vi "BCU诊断标定.vi"(8 "CAN端口":u16(ring), 9 "设备索引号":u16(ring), 10 "CAN卡类型":u32(ring)=21, 11 "Myindex":dbl=1.0) -> (3 "成功":bool)   [LabVIEW 2013] (continued)
                n1426 = global read "功能码全局.vi" "24"() -> (w1888:bool[])
                n1427 = global read "功能码全局.vi" "23"() -> (w1889:bool[])
                n1428 = Index Array(array=w1888) -> (element #3=w1878:bool, element #4=w1877:bool, element #5=w1876:bool, element #6=w1875:bool, element #7=w1874:bool, element #8=w1873:bool)  [unwired: 8 in, 2 out]
                n1429 = Index Array(array=w1889) -> (element #3=w1887:bool, element #4=w1886:bool, element #5=w1885:bool, element #6=w1884:bool, element #7=w1883:bool, element #8=w1882:bool)  [unwired: 8 in, 2 out]
                n1430 = Build Array(w1878, w1877, w1876, w1875, w1874, w1873) -> (w1879:bool[])
                n1431 = Build Array(w1887, w1886, w1885, w1884, w1883, w1882) -> (w1881:bool[])
                n1432 = And Array Elements(Boolean array=w1879) -> (logical AND=w1872:bool)
                n1433 = And Array Elements(Boolean array=w1881) -> (logical AND=w1880:bool)
                n1434 = Not(x=w1871) -> (.not. x?=w1895:bool)
              }
              frame "电池包信息1" {
                w1900 = 2
                w1908 = 2
                w1899 = 2
                w1897 = FALSE ("1 6")
                n1435 = Select(t=0, s=w1905, f=1) -> (s? t:f=w1898:i32)
                n1436 = property on="串联数" class="DigNum (严格)"("Disabled"=w1898) -> ()  [unwired: 2 in, 2 out]
                n1437 = property on="并联数" class="DigNum (严格)"("Disabled"=w1898) -> ()  [unwired: 2 in, 2 out]
                n1438 = property on="电池厂家" class="DigNum (严格)"("Disabled"=w1898) -> ()  [unwired: 2 in, 2 out]
                n1439 = property on="电池类型" class="DigNum (严格)"("Disabled"=w1898) -> ()  [unwired: 2 in, 2 out]
                n1440 = property on="额定能量" class="DigNum (严格)"("Disabled"=w1898) -> ()  [unwired: 2 in, 2 out]
                n1441 = property on="额定容量" class="DigNum (严格)"("Disabled"=w1898) -> ()  [unwired: 2 in, 2 out]
                n1442 = property on="实际容量" class="DigNum (严格)"("Disabled"=w1898) -> ()  [unwired: 2 in, 2 out]
                n1443 = property on="电池组信息" class="Clust (严格)"("Disabled"=w1898) -> ()  [unwired: 2 in, 2 out]
                n1444 = property on="生产日期" class="Str"("DisabledEnum"=w1898) -> ()  [unwired: 2 in, 2 out]
                n1445 = property on="车牌号" class="Str"("DisabledEnum"=w1899) -> ()  [unwired: 2 in, 2 out]
                n1446 = property on="产权标识" class="DigNum (严格)"("Disabled"=w1898) -> ()  [unwired: 2 in, 2 out]
                n1447 = property on="应用车型" class="DigNum (严格)"("Disabled"=w1898) -> ()  [unwired: 2 in, 2 out]
                n1448 = property on="额定总压" class="DigNum (严格)"("Disabled"=w1898) -> ()  [unwired: 2 in, 2 out]
                n1449 = property on="电池包序号" class="DigNum (严格)"("DisabledEnum"=w1898) -> ()  [unwired: 2 in, 2 out]
                n1450 = property on="电池包组号" class="DigNum (严格)"("DisabledEnum"=w1899) -> ()  [unwired: 2 in, 2 out]
                n1451 = property on="最大允许单体电压" class="DigNum (严格)"("Disabled"=w1908) -> ()  [unwired: 2 in, 2 out]
                n1452 = property on="最大允许总电压" class="DigNum (严格)"("Disabled"=w1908) -> ()  [unwired: 2 in, 2 out]
                n1453 = property on="最大允许温度" class="DigNum (严格)"("Disabled"=w1908) -> ()  [unwired: 2 in, 2 out]
                n1454 = property on="最小允许温度" class="DigNum (严格)"("Disabled"=w1908) -> ()  [unwired: 2 in, 2 out]
                n1455 = property on="最大允许充电电流" class="DigNum (严格)"("Disabled"=w1908) -> ()  [unwired: 2 in, 2 out]
                n1456 = property on="最小允许充电电流" class="DigNum (严格)"("Disabled"=w1908) -> ()  [unwired: 2 in, 2 out]
                n1457 = property on="最小允许单体电压" class="DigNum (严格)"("Disabled"=w1908) -> ()  [unwired: 2 in, 2 out]
                n1458 = property on="电流步长" class="DigNum (严格)"("Disabled"=w1908) -> ()  [unwired: 2 in, 2 out]
                n1459 = property on="SOC" class="DigNum (严格)"("Disabled"=w1908) -> ()  [unwired: 2 in, 2 out]
                n1460 = property on="充电总安时" class="DigNum (严格)"("Disabled"=w1908) -> ()  [unwired: 2 in, 2 out]
                n1461 = property on="放电总安时" class="DigNum (严格)"("Disabled"=w1908) -> ()  [unwired: 2 in, 2 out]
                n1462 = property on="放空次数" class="DigNum (严格)"("DisabledEnum"=w1900) -> ()  [unwired: 2 in, 2 out]
                n1463 = property on="充满次数" class="DigNum (严格)"("DisabledEnum"=w1900) -> ()  [unwired: 2 in, 2 out]
                n1464 = property on="充电次数" class="DigNum (严格)"("DisabledEnum"=w1900) -> ()  [unwired: 2 in, 2 out]
                n1465 = global read "功能码全局.vi" "24"() -> (w1903:bool[])
                n1466 = global read "功能码全局.vi" "23"() -> (w1904:bool[])
                n1467 = Index Array(array=w1903) -> (element #3=w1901:bool)  [unwired: 8 in, 7 out]
                n1468 = Index Array(array=w1904) -> (element #3=w1902:bool)  [unwired: 8 in, 7 out]
                n1469 = Not(x=w1897) -> (.not. x?=w1909:bool)
              }
              frame "电池包组号" {
                w1914 = 2
                w1913 = 2
                w1923 = 2
                w1915 = 2
                w1924 = 2
                w1911 = FALSE ("1 6")
                n1470 = property on="串联数" class="DigNum (严格)"("Disabled"=w1924) -> ()  [unwired: 2 in, 2 out]
                n1471 = property on="并联数" class="DigNum (严格)"("Disabled"=w1924) -> ()  [unwired: 2 in, 2 out]
                n1472 = property on="电池厂家" class="DigNum (严格)"("Disabled"=w1924) -> ()  [unwired: 2 in, 2 out]
                n1473 = property on="电池类型" class="DigNum (严格)"("Disabled"=w1924) -> ()  [unwired: 2 in, 2 out]
                n1474 = property on="额定能量" class="DigNum (严格)"("Disabled"=w1924) -> ()  [unwired: 2 in, 2 out]
                n1475 = property on="额定容量" class="DigNum (严格)"("Disabled"=w1924) -> ()  [unwired: 2 in, 2 out]
                n1476 = property on="实际容量" class="DigNum (严格)"("Disabled"=w1924) -> ()  [unwired: 2 in, 2 out]
                n1477 = Select(t=0, s=w1920, f=1) -> (s? t:f=w1912:i32)
                n1478 = property on="生产日期" class="Str"("DisabledEnum"=w1914) -> ()  [unwired: 2 in, 2 out]
                n1479 = property on="电池包序号" class="DigNum (严格)"("DisabledEnum"=w1914) -> ()  [unwired: 2 in, 2 out]
                n1480 = property on="车牌号" class="Str"("DisabledEnum"=w1914) -> ()  [unwired: 2 in, 2 out]
                n1481 = property on="电池包组号" class="DigNum (严格)"("DisabledEnum"=w1912) -> ()  [unwired: 2 in, 2 out]
                n1482 = property on="电池组信息" class="Clust (严格)"("Disabled"=w1912) -> ()  [unwired: 2 in, 2 out]
                n1483 = property on="产权标识" class="DigNum (严格)"("Disabled"=w1915) -> ()  [unwired: 2 in, 2 out]
                n1484 = property on="应用车型" class="DigNum (严格)"("Disabled"=w1915) -> ()  [unwired: 2 in, 2 out]
                n1485 = property on="额定总压" class="DigNum (严格)"("Disabled"=w1915) -> ()  [unwired: 2 in, 2 out]
                n1486 = property on="放空次数" class="DigNum (严格)"("DisabledEnum"=w1913) -> ()  [unwired: 2 in, 2 out]
                n1487 = property on="充满次数" class="DigNum (严格)"("DisabledEnum"=w1913) -> ()  [unwired: 2 in, 2 out]
                n1488 = property on="充电次数" class="DigNum (严格)"("DisabledEnum"=w1913) -> ()  [unwired: 2 in, 2 out]
                n1489 = property on="最大允许单体电压" class="DigNum (严格)"("Disabled"=w1923) -> ()  [unwired: 2 in, 2 out]
                n1490 = property on="最大允许总电压" class="DigNum (严格)"("Disabled"=w1923) -> ()  [unwired: 2 in, 2 out]
                n1491 = property on="最大允许温度" class="DigNum (严格)"("Disabled"=w1923) -> ()  [unwired: 2 in, 2 out]
                n1492 = property on="最小允许温度" class="DigNum (严格)"("Disabled"=w1923) -> ()  [unwired: 2 in, 2 out]
                n1493 = property on="最大允许充电电流" class="DigNum (严格)"("Disabled"=w1923) -> ()  [unwired: 2 in, 2 out]
                n1494 = property on="最小允许充电电流" class="DigNum (严格)"("Disabled"=w1923) -> ()  [unwired: 2 in, 2 out]
                n1495 = property on="最小允许单体电压" class="DigNum (严格)"("Disabled"=w1923) -> ()  [unwired: 2 in, 2 out]
                n1496 = property on="电流步长" class="DigNum (严格)"("Disabled"=w1923) -> ()  [unwired: 2 in, 2 out]
                n1497 = property on="SOC" class="DigNum (严格)"("Disabled"=w1923) -> ()  [unwired: 2 in, 2 out]
                n1498 = property on="充电总安时" class="DigNum (严格)"("Disabled"=w1923) -> ()  [unwired: 2 in, 2 out]
                n1499 = property on="放电总安时" class="DigNum (严格)"("Disabled"=w1923) -> ()  [unwired: 2 in, 2 out]
                n1500 = global read "功能码全局.vi" "24"() -> (w1918:bool[])
                n1501 = global read "功能码全局.vi" "23"() -> (w1919:bool[])
                n1502 = Index Array(array=w1918) -> (element #3=w1916:bool)  [unwired: 8 in, 7 out]
                n1503 = Index Array(array=w1919) -> (element #3=w1917:bool)  [unwired: 8 in, 7 out]
                n1504 = Not(x=w1911) -> (.not. x?=w1925:bool)
              }
              frame "充放电安时" {
                w1929 = 2
                w1928 = 2
                w1938 = 2
                w1939 = 2
                w1941 = 2
                w1927 = FALSE ("1 6")
                n1505 = property on="串联数" class="DigNum (严格)"("Disabled"=w1941) -> ()  [unwired: 2 in, 2 out]
                n1506 = property on="并联数" class="DigNum (严格)"("Disabled"=w1941) -> ()  [unwired: 2 in, 2 out]
                n1507 = property on="电池厂家" class="DigNum (严格)"("Disabled"=w1941) -> ()  [unwired: 2 in, 2 out]
                n1508 = property on="电池类型" class="DigNum (严格)"("Disabled"=w1941) -> ()  [unwired: 2 in, 2 out]
                n1509 = property on="额定能量" class="DigNum (严格)"("Disabled"=w1941) -> ()  [unwired: 2 in, 2 out]
                n1510 = property on="额定容量" class="DigNum (严格)"("Disabled"=w1941) -> ()  [unwired: 2 in, 2 out]
                n1511 = property on="实际容量" class="DigNum (严格)"("Disabled"=w1941) -> ()  [unwired: 2 in, 2 out]
                n1512 = Select(t=0, s=w1935, f=1) -> (s? t:f=w1934:i32)
                n1513 = property on="生产日期" class="Str"("DisabledEnum"=w1929) -> ()  [unwired: 2 in, 2 out]
                n1514 = property on="电池包序号" class="DigNum (严格)"("DisabledEnum"=w1929) -> ()  [unwired: 2 in, 2 out]
                n1515 = property on="车牌号" class="Str"("DisabledEnum"=w1929) -> ()  [unwired: 2 in, 2 out]
                n1516 = property on="电池包组号" class="DigNum (严格)"("DisabledEnum"=w1929) -> ()  [unwired: 2 in, 2 out]
                n1517 = property on="电池组信息" class="Clust (严格)"("Disabled"=w1934) -> ()  [unwired: 2 in, 2 out]
                n1518 = property on="额定总压" class="DigNum (严格)"("Disabled"=2) -> ()  [unwired: 2 in, 2 out]
                n1519 = property on="产权标识" class="DigNum (严格)"("Disabled"=w1939) -> ()  [unwired: 2 in, 2 out]
                n1520 = property on="应用车型" class="DigNum (严格)"("Disabled"=w1939) -> ()  [unwired: 2 in, 2 out]
                n1521 = property on="放空次数" class="DigNum (严格)"("DisabledEnum"=w1928) -> ()  [unwired: 2 in, 2 out]
                n1522 = property on="充满次数" class="DigNum (严格)"("DisabledEnum"=w1928) -> ()  [unwired: 2 in, 2 out]
                n1523 = property on="充电次数" class="DigNum (严格)"("DisabledEnum"=w1928) -> ()  [unwired: 2 in, 2 out]
                n1524 = property on="最大允许单体电压" class="DigNum (严格)"("Disabled"=w1938) -> ()  [unwired: 2 in, 2 out]
                n1525 = property on="最大允许总电压" class="DigNum (严格)"("Disabled"=w1938) -> ()  [unwired: 2 in, 2 out]
                n1526 = property on="最大允许温度" class="DigNum (严格)"("Disabled"=w1938) -> ()  [unwired: 2 in, 2 out]
                n1527 = property on="最小允许温度" class="DigNum (严格)"("Disabled"=w1938) -> ()  [unwired: 2 in, 2 out]
                n1528 = property on="最大允许充电电流" class="DigNum (严格)"("Disabled"=w1938) -> ()  [unwired: 2 in, 2 out]
                n1529 = property on="最小允许充电电流" class="DigNum (严格)"("Disabled"=w1938) -> ()  [unwired: 2 in, 2 out]
                n1530 = property on="最小允许单体电压" class="DigNum (严格)"("Disabled"=w1938) -> ()  [unwired: 2 in, 2 out]
                n1531 = property on="电流步长" class="DigNum (严格)"("Disabled"=w1938) -> ()  [unwired: 2 in, 2 out]
                n1532 = property on="SOC" class="DigNum (严格)"("Disabled"=w1938) -> ()  [unwired: 2 in, 2 out]
                n1533 = property on="充电总安时" class="DigNum (严格)"("Disabled"=w1934) -> ()  [unwired: 2 in, 2 out]
                n1534 = property on="放电总安时" class="DigNum (严格)"("Disabled"=w1934) -> ()  [unwired: 2 in, 2 out]
                n1535 = Not(x=w1927) -> (.not. x?=w1942:bool)
                n1536 = global read "功能码全局.vi" "24"() -> (w1932:bool[])
                n1537 = global read "功能码全局.vi" "23"() -> (w1933:bool[])
                n1538 = Index Array(array=w1932) -> (element #7=w1930:bool)  [unwired: 8 in, 7 out]
                n1539 = Index Array(array=w1933) -> (element #7=w1931:bool)  [unwired: 8 in, 7 out]
              }
              frame "充电次数" {
                w1947 = 2
                w1956 = 2
                w1957 = 2
                w1948 = 2
                w1958 = 2
                w1944 = FALSE ("1 6")
                n1540 = property on="串联数" class="DigNum (严格)"("Disabled"=w1958) -> ()  [unwired: 2 in, 2 out]
                n1541 = property on="并联数" class="DigNum (严格)"("Disabled"=w1958) -> ()  [unwired: 2 in, 2 out]
                n1542 = property on="电池厂家" class="DigNum (严格)"("Disabled"=w1958) -> ()  [unwired: 2 in, 2 out]
                n1543 = property on="电池类型" class="DigNum (严格)"("Disabled"=w1958) -> ()  [unwired: 2 in, 2 out]
                n1544 = property on="额定能量" class="DigNum (严格)"("Disabled"=w1958) -> ()  [unwired: 2 in, 2 out]
                n1545 = property on="额定容量" class="DigNum (严格)"("Disabled"=w1958) -> ()  [unwired: 2 in, 2 out]
                n1546 = property on="实际容量" class="DigNum (严格)"("Disabled"=w1958) -> ()  [unwired: 2 in, 2 out]
                n1547 = Select(t=0, s=w1953, f=1) -> (s? t:f=w1945:i32)
                n1548 = property on="生产日期" class="Str"("DisabledEnum"=w1947) -> ()  [unwired: 2 in, 2 out]
                n1549 = property on="电池包序号" class="DigNum (严格)"("DisabledEnum"=w1947) -> ()  [unwired: 2 in, 2 out]
                n1550 = property on="车牌号" class="Str"("DisabledEnum"=w1947) -> ()  [unwired: 2 in, 2 out]
                n1551 = property on="电池组信息" class="Clust (严格)"("Disabled"=w1945) -> ()  [unwired: 2 in, 2 out]
                n1552 = property on="电池包组号" class="DigNum (严格)"("DisabledEnum"=w1947) -> ()  [unwired: 2 in, 2 out]
                n1553 = property on="额定总压" class="DigNum (严格)"("Disabled"=w1948) -> ()  [unwired: 2 in, 2 out]
                n1554 = property on="产权标识" class="DigNum (严格)"("Disabled"=w1948) -> ()  [unwired: 2 in, 2 out]
                n1555 = property on="应用车型" class="DigNum (严格)"("Disabled"=w1948) -> ()  [unwired: 2 in, 2 out]
                n1556 = property on="放空次数" class="DigNum (严格)"("DisabledEnum"=w1945) -> (error out=w1946:errorcluster)  [unwired: 2 in, 1 out]
                n1557 = property on="充满次数" class="DigNum (严格)"("DisabledEnum"=w1945) -> ()  [unwired: 2 in, 2 out]
                n1558 = property on="充电次数" class="DigNum (严格)"("DisabledEnum"=w1945) -> ()  [unwired: 2 in, 2 out]
                n1559 = property on="最大允许单体电压" class="DigNum (严格)"("Disabled"=w1957) -> ()  [unwired: 2 in, 2 out]
                n1560 = property on="最大允许总电压" class="DigNum (严格)"("Disabled"=w1957) -> ()  [unwired: 2 in, 2 out]
                n1561 = property on="最大允许温度" class="DigNum (严格)"("Disabled"=w1957) -> ()  [unwired: 2 in, 2 out]
                n1562 = property on="最小允许温度" class="DigNum (严格)"("Disabled"=w1957) -> ()  [unwired: 2 in, 2 out]
                n1563 = property on="最大允许充电电流" class="DigNum (严格)"("Disabled"=w1957) -> ()  [unwired: 2 in, 2 out]
                n1564 = property on="最小允许充电电流" class="DigNum (严格)"(error in=w1946, "Disabled"=w1957) -> ()  [unwired: 1 in, 2 out]
                n1565 = property on="最小允许单体电压" class="DigNum (严格)"("Disabled"=w1957) -> ()  [unwired: 2 in, 2 out]
                n1566 = property on="电流步长" class="DigNum (严格)"("Disabled"=w1957) -> ()  [unwired: 2 in, 2 out]
                n1567 = property on="SOC" class="DigNum (严格)"("Disabled"=w1957) -> ()  [unwired: 2 in, 2 out]
                n1568 = property on="充电总安时" class="DigNum (严格)"("Disabled"=w1956) -> ()  [unwired: 2 in, 2 out]
                n1569 = property on="放电总安时" class="DigNum (严格)"("Disabled"=w1956) -> ()  [unwired: 2 in, 2 out]
                n1570 = Not(x=w1944) -> (.not. x?=w1959:bool)
                n1571 = global read "功能码全局.vi" "24"() -> (w1951:bool[])
                n1572 = global read "功能码全局.vi" "23"() -> (w1952:bool[])
                n1573 = Index Array(array=w1951) -> (element #8=w1950:bool)  [unwired: 8 in, 7 out]
                n1574 = Index Array(array=w1952) -> (element #8=w1949:bool)  [unwired: 8 in, 7 out]
              }
              frame "SOC" {
                w1963 = 2
                w1962 = 2
                w1972 = 2
                w1973 = 2
                w1974 = 2
                w1976 = 2
                w1961 = FALSE ("1 6")
                n1575 = property on="串联数" class="DigNum (严格)"("Disabled"=w1976) -> ()  [unwired: 2 in, 2 out]
                n1576 = property on="并联数" class="DigNum (严格)"("Disabled"=w1976) -> ()  [unwired: 2 in, 2 out]
                n1577 = property on="电池厂家" class="DigNum (严格)"("Disabled"=w1976) -> ()  [unwired: 2 in, 2 out]
                n1578 = property on="电池类型" class="DigNum (严格)"("Disabled"=w1976) -> ()  [unwired: 2 in, 2 out]
                n1579 = property on="额定能量" class="DigNum (严格)"("Disabled"=w1976) -> ()  [unwired: 2 in, 2 out]
                n1580 = property on="额定容量" class="DigNum (严格)"("Disabled"=w1976) -> ()  [unwired: 2 in, 2 out]
                n1581 = property on="实际容量" class="DigNum (严格)"("Disabled"=w1976) -> ()  [unwired: 2 in, 2 out]
                n1582 = Select(t=0, s=w1969, f=1) -> (s? t:f=w1968:i32)
                n1583 = property on="生产日期" class="Str"("DisabledEnum"=w1963) -> ()  [unwired: 2 in, 2 out]
                n1584 = property on="电池包序号" class="DigNum (严格)"("DisabledEnum"=w1963) -> ()  [unwired: 2 in, 2 out]
                n1585 = property on="车牌号" class="Str"("DisabledEnum"=w1963) -> ()  [unwired: 2 in, 2 out]
                n1586 = property on="电池包组号" class="DigNum (严格)"("DisabledEnum"=w1963) -> ()  [unwired: 2 in, 2 out]
                n1587 = property on="电池组信息" class="Clust (严格)"("Disabled"=w1968) -> ()  [unwired: 2 in, 2 out]
                n1588 = property on="SOC" class="DigNum (严格)"("Disabled"=w1968) -> ()  [unwired: 2 in, 2 out]
                n1589 = property on="额定总压" class="DigNum (严格)"("Disabled"=2) -> ()  [unwired: 2 in, 2 out]
                n1590 = property on="产权标识" class="DigNum (严格)"("Disabled"=w1974) -> ()  [unwired: 2 in, 2 out]
                n1591 = property on="应用车型" class="DigNum (严格)"("Disabled"=w1974) -> ()  [unwired: 2 in, 2 out]
                n1592 = property on="放空次数" class="DigNum (严格)"("DisabledEnum"=w1962) -> ()  [unwired: 2 in, 2 out]
                n1593 = property on="充满次数" class="DigNum (严格)"("DisabledEnum"=w1962) -> ()  [unwired: 2 in, 2 out]
                n1594 = property on="充电次数" class="DigNum (严格)"("DisabledEnum"=w1962) -> ()  [unwired: 2 in, 2 out]
                n1595 = property on="最大允许单体电压" class="DigNum (严格)"("Disabled"=w1973) -> ()  [unwired: 2 in, 2 out]
                n1596 = property on="最大允许总电压" class="DigNum (严格)"("Disabled"=w1973) -> ()  [unwired: 2 in, 2 out]
                n1597 = property on="最大允许温度" class="DigNum (严格)"("Disabled"=w1973) -> ()  [unwired: 2 in, 2 out]
                n1598 = property on="最小允许温度" class="DigNum (严格)"("Disabled"=w1973) -> ()  [unwired: 2 in, 2 out]
                n1599 = property on="最大允许充电电流" class="DigNum (严格)"("Disabled"=w1973) -> ()  [unwired: 2 in, 2 out]
                n1600 = property on="最小允许充电电流" class="DigNum (严格)"("Disabled"=w1973) -> ()  [unwired: 2 in, 2 out]
                n1601 = property on="最小允许单体电压" class="DigNum (严格)"("Disabled"=w1973) -> ()  [unwired: 2 in, 2 out]
                n1602 = property on="电流步长" class="DigNum (严格)"("Disabled"=w1973) -> ()  [unwired: 2 in, 2 out]
                n1603 = property on="充电总安时" class="DigNum (严格)"("Disabled"=w1972) -> ()  [unwired: 2 in, 2 out]
                n1604 = property on="放电总安时" class="DigNum (严格)"("Disabled"=w1972) -> ()  [unwired: 2 in, 2 out]
                n1605 = Not(x=w1961) -> (.not. x?=w1977:bool)
                n1606 = global read "功能码全局.vi" "24"() -> (w1966:bool[])
                n1607 = global read "功能码全局.vi" "23"() -> (w1967:bool[])
                n1608 = Index Array(array=w1966) -> (element #6=w1965:bool)  [unwired: 8 in, 7 out]
                n1609 = Index Array(array=w1967) -> (element #6=w1964:bool)  [unwired: 8 in, 7 out]
              }
              frame "车牌号" {
                w1982 = 2
                w1981 = 2
                w1991 = 2
                w1992 = 2
                w1993 = 2
                w1995 = 2
                w1979 = FALSE ("1 6")
                n1610 = property on="串联数" class="DigNum (严格)"("Disabled"=w1995) -> ()  [unwired: 2 in, 2 out]
                n1611 = property on="并联数" class="DigNum (严格)"("Disabled"=w1995) -> ()  [unwired: 2 in, 2 out]
                n1612 = property on="电池厂家" class="DigNum (严格)"("Disabled"=w1995) -> ()  [unwired: 2 in, 2 out]
                n1613 = property on="电池类型" class="DigNum (严格)"("Disabled"=w1995) -> ()  [unwired: 2 in, 2 out]
                n1614 = property on="额定能量" class="DigNum (严格)"("Disabled"=w1995) -> ()  [unwired: 2 in, 2 out]
                n1615 = property on="额定容量" class="DigNum (严格)"("Disabled"=w1995) -> ()  [unwired: 2 in, 2 out]
                n1616 = property on="实际容量" class="DigNum (严格)"("Disabled"=w1995) -> ()  [unwired: 2 in, 2 out]
                n1617 = Select(t=0, s=w1987, f=1) -> (s? t:f=w1980:i32)
                n1618 = property on="生产日期" class="Str"("DisabledEnum"=w1982) -> ()  [unwired: 2 in, 2 out]
                n1619 = property on="电池包序号" class="DigNum (严格)"("DisabledEnum"=w1982) -> ()  [unwired: 2 in, 2 out]
                n1620 = property on="电池包组号" class="DigNum (严格)"("DisabledEnum"=w1982) -> ()  [unwired: 2 in, 2 out]
                n1621 = property on="电池组信息" class="Clust (严格)"("Disabled"=w1980) -> ()  [unwired: 2 in, 2 out]
                n1622 = property on="车牌号" class="Str"("DisabledEnum"=w1980) -> ()  [unwired: 2 in, 2 out]
                n1623 = property on="额定总压" class="DigNum (严格)"("Disabled"=2) -> ()  [unwired: 2 in, 2 out]
                n1624 = property on="产权标识" class="DigNum (严格)"("Disabled"=w1993) -> ()  [unwired: 2 in, 2 out]
                n1625 = property on="应用车型" class="DigNum (严格)"("Disabled"=w1993) -> ()  [unwired: 2 in, 2 out]
                n1626 = property on="放空次数" class="DigNum (严格)"("DisabledEnum"=w1981) -> ()  [unwired: 2 in, 2 out]
                n1627 = property on="充满次数" class="DigNum (严格)"("DisabledEnum"=w1981) -> ()  [unwired: 2 in, 2 out]
                n1628 = property on="充电次数" class="DigNum (严格)"("DisabledEnum"=w1981) -> ()  [unwired: 2 in, 2 out]
                n1629 = property on="最大允许单体电压" class="DigNum (严格)"("Disabled"=w1992) -> ()  [unwired: 2 in, 2 out]
                n1630 = property on="最大允许总电压" class="DigNum (严格)"("Disabled"=w1992) -> ()  [unwired: 2 in, 2 out]
                n1631 = property on="最大允许温度" class="DigNum (严格)"("Disabled"=w1992) -> ()  [unwired: 2 in, 2 out]
                n1632 = property on="最小允许温度" class="DigNum (严格)"("Disabled"=w1992) -> ()  [unwired: 2 in, 2 out]
                n1633 = property on="最大允许充电电流" class="DigNum (严格)"("Disabled"=w1992) -> ()  [unwired: 2 in, 2 out]
                n1634 = property on="最小允许充电电流" class="DigNum (严格)"("Disabled"=w1992) -> ()  [unwired: 2 in, 2 out]
                n1635 = property on="最小允许单体电压" class="DigNum (严格)"("Disabled"=w1992) -> ()  [unwired: 2 in, 2 out]
                n1636 = property on="电流步长" class="DigNum (严格)"("Disabled"=w1992) -> ()  [unwired: 2 in, 2 out]
                n1637 = property on="SOC" class="DigNum (严格)"("Disabled"=2) -> ()  [unwired: 2 in, 2 out]
                n1638 = property on="充电总安时" class="DigNum (严格)"("Disabled"=w1991) -> ()  [unwired: 2 in, 2 out]
                n1639 = property on="放电总安时" class="DigNum (严格)"("Disabled"=w1991) -> ()  [unwired: 2 in, 2 out]
                n1640 = Not(x=w1979) -> (.not. x?=w1996:bool)
                n1641 = global read "功能码全局.vi" "24"() -> (w1985:bool[])
                n1642 = global read "功能码全局.vi" "23"() -> (w1986:bool[])
                n1643 = Index Array(array=w1985) -> (element #5=w1983:bool)  [unwired: 8 in, 7 out]
                n1644 = Index Array(array=w1986) -> (element #5=w1984:bool)  [unwired: 8 in, 7 out]
              }
              frame "充电参数" {
                w2000 = 2
                w1999 = 2
                w2009 = 2
                w2010 = 2
                w2012 = 2
                w1998 = FALSE ("1 6")
                n1645 = property on="串联数" class="DigNum (严格)"("Disabled"=w2012) -> ()  [unwired: 2 in, 2 out]
                n1646 = property on="并联数" class="DigNum (严格)"("Disabled"=w2012) -> ()  [unwired: 2 in, 2 out]
                n1647 = property on="电池厂家" class="DigNum (严格)"("Disabled"=w2012) -> ()  [unwired: 2 in, 2 out]
                n1648 = property on="电池类型" class="DigNum (严格)"("Disabled"=w2012) -> ()  [unwired: 2 in, 2 out]
                n1649 = property on="额定能量" class="DigNum (严格)"("Disabled"=w2012) -> ()  [unwired: 2 in, 2 out]
                n1650 = property on="额定容量" class="DigNum (严格)"("Disabled"=w2012) -> ()  [unwired: 2 in, 2 out]
                n1651 = property on="实际容量" class="DigNum (严格)"("Disabled"=w2012) -> ()  [unwired: 2 in, 2 out]
                n1652 = Select(t=0, s=w2006, f=1) -> (s? t:f=w2005:i32)
                n1653 = property on="生产日期" class="Str"("DisabledEnum"=w2000) -> ()  [unwired: 2 in, 2 out]
                n1654 = property on="电池包序号" class="DigNum (严格)"("DisabledEnum"=w2000) -> ()  [unwired: 2 in, 2 out]
                n1655 = property on="车牌号" class="Str"("DisabledEnum"=w2000) -> ()  [unwired: 2 in, 2 out]
                n1656 = property on="电池组信息" class="Clust (严格)"("Disabled"=w2005) -> ()  [unwired: 2 in, 2 out]
                n1657 = property on="电池包组号" class="DigNum (严格)"("DisabledEnum"=w2000) -> ()  [unwired: 2 in, 2 out]
                n1658 = property on="额定总压" class="DigNum (严格)"("Disabled"=2) -> ()  [unwired: 2 in, 2 out]
                n1659 = property on="产权标识" class="DigNum (严格)"("Disabled"=w2010) -> ()  [unwired: 2 in, 2 out]
                n1660 = property on="应用车型" class="DigNum (严格)"("Disabled"=w2010) -> ()  [unwired: 2 in, 2 out]
                n1661 = property on="放空次数" class="DigNum (严格)"("DisabledEnum"=w1999) -> ()  [unwired: 2 in, 2 out]
                n1662 = property on="充满次数" class="DigNum (严格)"("DisabledEnum"=w1999) -> ()  [unwired: 2 in, 2 out]
                n1663 = property on="充电次数" class="DigNum (严格)"("DisabledEnum"=w1999) -> ()  [unwired: 2 in, 2 out]
                n1664 = property on="最大允许单体电压" class="DigNum (严格)"("Disabled"=w2005) -> ()  [unwired: 2 in, 2 out]
                n1665 = property on="最大允许总电压" class="DigNum (严格)"("Disabled"=w2005) -> ()  [unwired: 2 in, 2 out]
                n1666 = property on="最大允许温度" class="DigNum (严格)"("Disabled"=w2005) -> ()  [unwired: 2 in, 2 out]
                n1667 = property on="最小允许温度" class="DigNum (严格)"("Disabled"=w2005) -> ()  [unwired: 2 in, 2 out]
                n1668 = property on="最大允许充电电流" class="DigNum (严格)"("Disabled"=w2005) -> ()  [unwired: 2 in, 2 out]
                n1669 = property on="最小允许充电电流" class="DigNum (严格)"("Disabled"=w2005) -> ()  [unwired: 2 in, 2 out]
                n1670 = property on="最小允许单体电压" class="DigNum (严格)"("Disabled"=w2005) -> ()  [unwired: 2 in, 2 out]
                n1671 = property on="电流步长" class="DigNum (严格)"("Disabled"=w2005) -> ()  [unwired: 2 in, 2 out]
                n1672 = property on="SOC" class="DigNum (严格)"("Disabled"=w2009) -> ()  [unwired: 2 in, 2 out]
                n1673 = property on="充电总安时" class="DigNum (严格)"("Disabled"=w2009) -> ()  [unwired: 2 in, 2 out]
                n1674 = property on="放电总安时" class="DigNum (严格)"("Disabled"=w2009) -> ()  [unwired: 2 in, 2 out]
                n1675 = Not(x=w1998) -> (.not. x?=w2013:bool)
                n1676 = global read "功能码全局.vi" "24"() -> (w2003:bool[])
                n1677 = global read "功能码全局.vi" "23"() -> (w2004:bool[])
                n1678 = Index Array(array=w2003) -> (element #4=w2001:bool)  [unwired: 8 in, 7 out]
                n1679 = Index Array(array=w2004) -> (element #4=w2002:bool)  [unwired: 8 in, 7 out]
              }
              frame "均衡参数" {
                w2015 = FALSE ("1 6")
                n1680 = Select(t=0, s=w2021, f=1) -> (s? t:f=w2019:i32)
                n1681 = property on="均衡计算-电压高阀值1级" class="DigNum (严格)"("DisabledEnum"=w2019) -> ()  [unwired: 2 in, 2 out]
                n1682 = property on="均衡计算-电压高阀值2级" class="DigNum (严格)"("DisabledEnum"=w2019) -> ()  [unwired: 2 in, 2 out]
                n1683 = property on="均衡计算-电压低阀值1级" class="DigNum (严格)"("DisabledEnum"=w2019) -> ()  [unwired: 2 in, 2 out]
                n1684 = property on="均衡计算-电压低阀值2级" class="DigNum (严格)"("DisabledEnum"=w2019) -> ()  [unwired: 2 in, 2 out]
                n1685 = property on="均衡计算-最低电压阀值" class="DigNum (严格)"("DisabledEnum"=w2019) -> ()  [unwired: 2 in, 2 out]
                n1686 = property on="均衡停止-最低电压阀值" class="DigNum (严格)"("DisabledEnum"=w2019) -> ()  [unwired: 2 in, 2 out]
                n1687 = property on="均衡计算-电压极差阀值" class="DigNum (严格)"("DisabledEnum"=w2019) -> ()  [unwired: 2 in, 2 out]
                n1688 = property on="均衡参数" class="Clust (严格)"("DisabledEnum"=w2019) -> ()  [unwired: 2 in, 2 out]
                n1689 = property on="充电结束电压(90%)" class="DigNum (严格)"("DisabledEnum"=w2019) -> ()  [unwired: 2 in, 2 out]
                n1690 = property on="充电结束电压(91%)" class="DigNum (严格)"("DisabledEnum"=w2019) -> ()  [unwired: 2 in, 2 out]
                n1691 = property on="充电结束电压(92%)" class="DigNum (严格)"("DisabledEnum"=w2019) -> ()  [unwired: 2 in, 2 out]
                n1692 = property on="充电结束电压(93%)" class="DigNum (严格)"("DisabledEnum"=w2019) -> ()  [unwired: 2 in, 2 out]
                n1693 = property on="充电结束电压(94%)" class="DigNum (严格)"("DisabledEnum"=w2019) -> ()  [unwired: 2 in, 2 out]
                n1694 = property on="充电结束电压(95%)" class="DigNum (严格)"("DisabledEnum"=w2019) -> ()  [unwired: 2 in, 2 out]
                n1695 = property on="充电结束电压(96%)" class="DigNum (严格)"("DisabledEnum"=w2019) -> ()  [unwired: 2 in, 2 out]
                n1696 = property on="充电结束电压(97%)" class="DigNum (严格)"("DisabledEnum"=w2019) -> ()  [unwired: 2 in, 2 out]
                n1697 = property on="充电结束电压(98%)" class="DigNum (严格)"("DisabledEnum"=w2019) -> ()  [unwired: 2 in, 2 out]
                n1698 = property on="充电结束电压(99%)" class="DigNum (严格)"("DisabledEnum"=w2019) -> ()  [unwired: 2 in, 2 out]
                n1699 = property on="充电结束电压(100%)" class="DigNum (严格)"("DisabledEnum"=w2019) -> ()  [unwired: 2 in, 2 out]
                n1700 = disable-structure shown="启用" {
                  disable-tunnel: [w2025 w2027] -> w2018
                  disable-tunnel: [w2024 w2027] -> w2017
                  frame Enabled {
                    n1701 = global read "功能码全局.vi" "18"() -> (w2026:bool[])
                    n1702 = Index Array(array=w2026) -> (element #1=w2025:bool, element #2=w2024:bool)  [unwired: 8 in, 6 out]
                  }
                  frame Disabled {
                    w2027 = TRUE
                  }
                }
                n1703 = Not(x=w2015) -> (.not. x?=w2016:bool)
              }
              frame "均衡阀值" {
                w2030 = 2
                w2028 = FALSE ("1 6")
                n1704 = Select(t=0, s=w2035, f=1) -> (s? t:f=w2033:i32)
                n1705 = property on="均衡计算-电压高阀值1级" class="DigNum (严格)"("DisabledEnum"=w2033) -> ()  [unwired: 2 in, 2 out]
                n1706 = property on="均衡计算-电压高阀值2级" class="DigNum (严格)"("DisabledEnum"=w2033) -> ()  [unwired: 2 in, 2 out]
                n1707 = property on="均衡计算-电压低阀值1级" class="DigNum (严格)"("DisabledEnum"=w2033) -> ()  [unwired: 2 in, 2 out]
                n1708 = property on="均衡计算-电压低阀值2级" class="DigNum (严格)"("DisabledEnum"=w2033) -> ()  [unwired: 2 in, 2 out]
                n1709 = property on="均衡计算-最低电压阀值" class="DigNum (严格)"("DisabledEnum"=w2033) -> ()  [unwired: 2 in, 2 out]
                n1710 = property on="均衡停止-最低电压阀值" class="DigNum (严格)"("DisabledEnum"=w2033) -> ()  [unwired: 2 in, 2 out]
                n1711 = property on="均衡计算-电压极差阀值" class="DigNum (严格)"("DisabledEnum"=w2033) -> ()  [unwired: 2 in, 2 out]
                n1712 = property on="均衡参数" class="Clust (严格)"("DisabledEnum"=w2033) -> ()  [unwired: 2 in, 2 out]
                n1713 = property on="充电结束电压(90%)" class="DigNum (严格)"("DisabledEnum"=w2030) -> ()  [unwired: 2 in, 2 out]
                n1714 = property on="充电结束电压(91%)" class="DigNum (严格)"("DisabledEnum"=w2030) -> ()  [unwired: 2 in, 2 out]
                n1715 = property on="充电结束电压(92%)" class="DigNum (严格)"("DisabledEnum"=w2030) -> ()  [unwired: 2 in, 2 out]
                n1716 = property on="充电结束电压(93%)" class="DigNum (严格)"("DisabledEnum"=w2030) -> ()  [unwired: 2 in, 2 out]
                n1717 = property on="充电结束电压(94%)" class="DigNum (严格)"("DisabledEnum"=w2030) -> ()  [unwired: 2 in, 2 out]
                n1718 = property on="充电结束电压(95%)" class="DigNum (严格)"("DisabledEnum"=w2030) -> ()  [unwired: 2 in, 2 out]
                n1719 = property on="充电结束电压(96%)" class="DigNum (严格)"("DisabledEnum"=w2030) -> ()  [unwired: 2 in, 2 out]
                n1720 = property on="充电结束电压(97%)" class="DigNum (严格)"("DisabledEnum"=w2030) -> ()  [unwired: 2 in, 2 out]
                n1721 = property on="充电结束电压(98%)" class="DigNum (严格)"("DisabledEnum"=w2030) -> ()  [unwired: 2 in, 2 out]
                n1722 = property on="充电结束电压(99%)" class="DigNum (严格)"("DisabledEnum"=w2030) -> ()  [unwired: 2 in, 2 out]
                n1723 = property on="充电结束电压(100%)" class="DigNum (严格)"("DisabledEnum"=w2030) -> ()  [unwired: 2 in, 2 out]
                n1724 = disable-structure shown="启用" {
                  disable-tunnel: [w2039 w2041] -> w2032
                  disable-tunnel: [w2038 w2041] -> w2031
                  frame Enabled {
                    n1725 = global read "功能码全局.vi" "18"() -> (w2040:bool[])
                    n1726 = Index Array(array=w2040) -> (element #1=w2039:bool, element #2=w2038:bool)  [unwired: 8 in, 6 out]
                  }
                  frame Disabled {
                    w2041 = TRUE
                  }
                }
                n1727 = Not(x=w2028) -> (.not. x?=w2029:bool)
              }
              frame "充电结束电压" {
                w2045 = 2
                w2042 = FALSE ("1 6")
                n1728 = Select(t=0, s=w2049, f=1) -> (s? t:f=w2044:i32)
                n1729 = property on="均衡计算-电压高阀值1级" class="DigNum (严格)"("DisabledEnum"=w2045) -> ()  [unwired: 2 in, 2 out]
                n1730 = property on="均衡计算-电压高阀值2级" class="DigNum (严格)"("DisabledEnum"=w2045) -> ()  [unwired: 2 in, 2 out]
                n1731 = property on="均衡计算-电压低阀值1级" class="DigNum (严格)"("DisabledEnum"=w2045) -> ()  [unwired: 2 in, 2 out]
                n1732 = property on="均衡计算-电压低阀值2级" class="DigNum (严格)"("DisabledEnum"=w2045) -> ()  [unwired: 2 in, 2 out]
                n1733 = property on="均衡计算-最低电压阀值" class="DigNum (严格)"("DisabledEnum"=w2045) -> ()  [unwired: 2 in, 2 out]
                n1734 = property on="均衡停止-最低电压阀值" class="DigNum (严格)"("DisabledEnum"=w2045) -> ()  [unwired: 2 in, 2 out]
                n1735 = property on="均衡计算-电压极差阀值" class="DigNum (严格)"("DisabledEnum"=w2045) -> ()  [unwired: 2 in, 2 out]
                n1736 = property on="均衡参数" class="Clust (严格)"("DisabledEnum"=w2044) -> ()  [unwired: 2 in, 2 out]
                n1737 = property on="充电结束电压(90%)" class="DigNum (严格)"("DisabledEnum"=w2044) -> ()  [unwired: 2 in, 2 out]
                n1738 = property on="充电结束电压(91%)" class="DigNum (严格)"("DisabledEnum"=w2044) -> ()  [unwired: 2 in, 2 out]
                n1739 = property on="充电结束电压(92%)" class="DigNum (严格)"("DisabledEnum"=w2044) -> ()  [unwired: 2 in, 2 out]
                n1740 = property on="充电结束电压(93%)" class="DigNum (严格)"("DisabledEnum"=w2044) -> ()  [unwired: 2 in, 2 out]
                n1741 = property on="充电结束电压(94%)" class="DigNum (严格)"("DisabledEnum"=w2044) -> ()  [unwired: 2 in, 2 out]
                n1742 = property on="充电结束电压(95%)" class="DigNum (严格)"("DisabledEnum"=w2044) -> ()  [unwired: 2 in, 2 out]
                n1743 = property on="充电结束电压(96%)" class="DigNum (严格)"("DisabledEnum"=w2044) -> ()  [unwired: 2 in, 2 out]
                n1744 = property on="充电结束电压(97%)" class="DigNum (严格)"("DisabledEnum"=w2044) -> ()  [unwired: 2 in, 2 out]
                n1745 = property on="充电结束电压(98%)" class="DigNum (严格)"("DisabledEnum"=w2044) -> ()  [unwired: 2 in, 2 out]
                n1746 = property on="充电结束电压(99%)" class="DigNum (严格)"("DisabledEnum"=w2044) -> ()  [unwired: 2 in, 2 out]
                n1747 = property on="充电结束电压(100%)" class="DigNum (严格)"("DisabledEnum"=w2044) -> ()  [unwired: 2 in, 2 out]
                n1748 = disable-structure shown="启用" {
                  disable-tunnel: [w2053 w2055] -> w2047
                  disable-tunnel: [w2052 w2055] -> w2046
                  frame Enabled {
                    n1749 = global read "功能码全局.vi" "18"() -> (w2054:bool[])
                    n1750 = Index Array(array=w2054) -> (element #1=w2053:bool, element #2=w2052:bool)  [unwired: 8 in, 6 out]
                  }
                  frame Disabled {
                    w2055 = TRUE
                  }
                }
                n1751 = Not(x=w2042) -> (.not. x?=w2043:bool)
              }
              frame "假", Default {
                w2056 = FALSE ("1 6")
                n1752 = Not(x=w2056) -> (.not. x?=w2057:bool)
              }
            }
            n1753 = local write "等级 2"(w1647) -> ()
            n1754 = local write "1 6"(w1646) -> ()
            n1755 = local write "1 7"(w1645) -> ()
            n1756 = local write "1 8"(w1644) -> ()
            n1757 = local write "1 9"(w1643) -> ()
            n1758 = local write "1 10"(w1642) -> ()
            n1759 = local write "1 12"(w1636) -> ()
            n1760 = property on="单个读取" class="Bool (严格)"("Visible"=w1641) -> ()  [unwired: 2 in, 2 out]
            n1761 = property on="单个写入" class="Bool (严格)"("Visible"=w1640) -> ()  [unwired: 2 in, 2 out]
          }
          event "从板个数": Value Change {
            n1762 = event-data() -> ()  [unwired: 7 out]
            n1763 = local read "从板个数"() -> (w2059:dbl)
            n1764 = call "多从板对应参数-new.vi"("从板个数"=w2059) -> ("输出数组"=w2060:string[])  [unwired: 1 in]
            n1765 = control-ref of="项目信息"() -> (w2061:refnum<vi>)
            n1766 = stacked-sequence {
              tunnel: w2061 -> [_ w2068 w2072]
              tunnel: w2060 -> [_ w2067 w2071]
              frame #0 {
                n1767 = local write "项目信息"(string[][] [] ("项目信息")) -> ()
              }
              frame #1 {
                n1768 = call "表格数据输入-8.6.vi"("行数"=u32 0, "列数"=u32 0, "字符串数组"=w2067, "表格引用"=w2068) -> ()  [unwired: 8 out]
              }
              frame #2 {
                n1769 = Array Size(array=w2071) -> (size(s)=w2070:i32)
                n1770 = for {
                  N: w2070 -> [_]
                  tunnel: [""] -> w2069 mode=indexing
                }
                n1771 = call "表格数据输入-8.6.vi"("行数"=u32 0, "列数"=u32 1, "字符串数组"=w2069, "表格引用"=w2072) -> ()  [unwired: 8 out]
              }
            }
          }
          event "主界面选项": Value Change {
            n1772 = event-data() -> ("NewVal"=w2076:enum32{"单选选项1", "单选选项2", "单选选项2 2", "单选选项2 3"})  [unwired: 6 out]
            n1773 = control-ref of="单选选项2 2"() -> (w2081:refnum<vi>)
            n1774 = control-ref of="单选选项2"() -> (w2083:refnum<vi>)
            n1775 = control-ref of="单选选项1"() -> (w2082:refnum<vi>)
            n1776 = control-ref of="单选选项2 3"() -> (w2077:refnum<vi>)
            n1777 = Build Array(w2082, w2083, w2081, w2077) -> (w2080:refnum<vi>[])
            n1778 = case shown="\"单选选项2 3\"" w2076 {
              selector: w2076 -> [w2094 w2099 w2104 w2109]
              tunnel: w2080 -> [w2095 w2100 w2105 w2110]
              tunnel: [w2093 w2098 w2103 w2108] -> w2086
              tunnel: [w2092 w2097 w2102 w2107] -> w2085
              tunnel: [enum32{"读写参数", "版本读取", "其它诊断"}."读写参数" ("选项卡控件 2") enum32{"读写参数", "版本读取", "其它诊断"}."版本读取" ("选项卡控件 2") enum32{"读写参数", "版本读取", "其它诊断"}."其它诊断" ("选项卡控件 2") enum32{"读写参数", "版本读取", "其它诊断", "高压板校正"}."高压板校正" ("选项卡控件 2")] -> w2084
              frame "单选选项1", Default {
                n1779 = Delete From Array(array=w2095, index=w2094) -> (deleted portion=w2092:refnum<vi>, array with subset deleted=w2093:refnum<vi>[])  [unwired: 1 in]
              }
              frame "单选选项2" {
                n1780 = Delete From Array(array=w2100, index=w2099) -> (deleted portion=w2097:refnum<vi>, array with subset deleted=w2098:refnum<vi>[])  [unwired: 1 in]
              }
              frame "单选选项2 2" {
                n1781 = Delete From Array(array=w2105, index=w2104) -> (deleted portion=w2102:refnum<vi>, array with subset deleted=w2103:refnum<vi>[])  [unwired: 1 in]
              }
              frame "单选选项2 3" {
                n1782 = Delete From Array(array=w2110, index=w2109) -> (deleted portion=w2107:refnum<vi>, array with subset deleted=w2108:refnum<vi>[])  [unwired: 1 in]
              }
            }
            n1783 = local write "面板选择"(w2084) -> ()
            n1784 = for {
              tunnel: u32 16777215 -> [w2090]
              tunnel: w2086 -> [w2089] mode=indexing
              n1785 = property class="Bool (严格)"(reference=w2089, "BoolText.TextColor"=w2090) -> ()  [unwired: 1 in, 2 out]
            }
            n1786 = property class="Bool (严格)"(reference=w2085, "BoolText.TextColor"=u32 65511) -> ()  [unwired: 1 in, 2 out]
          }
          event "主从板": Value Change {
            w2112 = FALSE ("可见")
            n1787 = event-data() -> ()  [unwired: 7 out]
            n1788 = control-ref of="单选选项2"() -> (w2120:refnum<vi>)
            n1789 = control-ref of="单选选项1"() -> (w2119:refnum<vi>)
            n1790 = local read "主从板"() -> (w2127:enum32{"单选选项2", "单选选项1"})
            n1791 = Build Array(w2120, w2119) -> (w2126:refnum<vi>[])
            n1792 = case shown="\"单选选项2\"" w2127 {
              selector: w2127 -> [w2172 w2215]
              tunnel: w2126 -> [w2173 w2214]
              tunnel: [enum32{"主板", "从板"}."主板" ("主从选择") enum32{"主板", "从板"}."从板" ("主从选择")] -> w2125
              tunnel: [w2171 w2213] -> w2122
              tunnel: [w2170 w2212] -> w2121
              tunnel: [TRUE FALSE] -> w2117
              tunnel: [w2131 w2192] -> w2114
              tunnel: [w2132 w2197] -> w2113
              tunnel: [FALSE ("可见") TRUE ("可见")] -> w2111
              frame "单选选项1", Default {
                n1793 = global read "功能码全局.vi" "主板项目信息7"() -> (w2143:bool[])
                n1794 = global read "功能码全局.vi" "主板项目信息4"() -> (w2166:bool[])
                n1795 = global read "功能码全局.vi" "主板控制类信息10"() -> (w2147:bool[])
                n1796 = global read "功能码全局.vi" "主板故障阀值9"() -> (w2144:bool[])
                n1797 = global read "功能码全局.vi" "主板项目信息5"() -> (w2157:bool[])
                n1798 = global read "功能码全局.vi" "主板项目信息6"() -> (w2167:bool[])
                n1799 = global read "功能码全局.vi" "主板版本号11"() -> (w2158:bool[])
                n1800 = Delete From Array(array=w2167, length=1 ("长度"), index=0 ("索引")) -> (deleted portion=w2156:bool[], array with subset deleted=w2139:bool[])
                n1801 = Index Array(array=w2166, index #1=5 ("索引"), index #2=6 ("索引")) -> (element #1=w2155:bool, element #2=w2138:bool)
                n1802 = Index Array(array=w2158) -> (element #1=w2151:bool, element #2=w2134:bool)  [unwired: 2 in]
                n1803 = Array Subset(array=w2144, index=2 ("索引"), length=3 ("长度")) -> (w2153:bool[])
                n1804 = Delete From Array(array=w2143, length=3 ("索引"), index=2 ("长度")) -> (deleted portion=w2154:bool[], array with subset deleted=w2137:bool[])
                n1805 = Array Subset(array=w2147, index=4 ("索引"), length=2 ("长度")) -> (w2152:bool[])
                n1806 = Delete From Array(array=w2173, index=w2172) -> (deleted portion=w2170:refnum<vi>, array with subset deleted=w2171:refnum<vi>[])  [unwired: 1 in]
                n1807 = Insert Into Array(array=w2157, new element #1=w2156, new element #2=w2155, new element #3=w2154, new element #4=w2153, new element #5=w2152, new element #6=w2151) -> (w2150:bool[])  [unwired: 1 in]
                n1808 = Array Subset(array=w2147, index=6 ("索引"), length=2 ("长度")) -> (w2135:bool[])
                n1809 = Array Subset(array=w2144, index=5 ("索引"), length=3 ("长度")) -> (w2136:bool[])
                n1810 = And Array Elements(Boolean array=w2150) -> (logical AND=w2132:bool)
                n1811 = Insert Into Array(array=w2139, new element #1=w2138, new element #2=w2137, new element #3=w2136, new element #4=w2135, new element #5=w2134) -> (w2133:bool[])  [unwired: 1 in]
                n1812 = And Array Elements(Boolean array=w2133) -> (logical AND=w2131:bool)
              }
              frame "单选选项2" {
                n1813 = global read "功能码全局.vi" "18"() -> (w2188:bool[])
                n1814 = global read "功能码全局.vi" "15"() -> (w2209:bool[])
                n1815 = global read "功能码全局.vi" "16"() -> (w2206:bool[])
                n1816 = Delete From Array(array=w2214, index=w2215) -> (deleted portion=w2212:refnum<vi>, array with subset deleted=w2213:refnum<vi>[])  [unwired: 1 in]
                n1817 = Index Array(array=w2206, index #1=4 ("索引"), index #2=5 ("索引"), index #3=6 ("索引"), index #4=7 ("索引")) -> (element #1=w2200:bool, element #2=w2199:bool, element #3=w2195:bool, element #4=w2194:bool)
                n1818 = Index Array(array=w2188, index #1=4 ("索引"), index #2=5 ("索引"), index #3=6 ("索引"), index #4=7 ("索引"), index #5=2 ("索引"), index #6=3 ("索引"), index #7=0 ("索引"), index #8=1 ("索引")) -> (element #1=w2181:bool, element #2=w2184:bool, element #3=w2183:bool, element #4=w2182:bool, element #5=w2180:bool, element #6=w2179:bool, element #7=w2174:bool, element #8=w2175:bool)
                n1819 = Delete From Array(array=w2209, length=4 ("长度"), index=0 ("索引")) -> (deleted portion=w2201:bool[], array with subset deleted=w2196:bool[])
                n1820 = Insert Into Array(array=w2196, new element #1=w2195, new element #2=w2194, new element #3=w2184, new element #4=w2183, new element #5=w2182, new element #6=w2175) -> (w2193:bool[])  [unwired: 1 in]
                n1821 = Insert Into Array(array=w2201, new element #1=w2200, new element #2=w2199, new element #3=w2181, new element #4=w2180, new element #5=w2179, new element #6=w2174) -> (w2198:bool[])  [unwired: 1 in]
                n1822 = And Array Elements(Boolean array=w2198) -> (logical AND=w2197:bool)
                n1823 = And Array Elements(Boolean array=w2193) -> (logical AND=w2192:bool)
              }
            }
            n1824 = property on="全部写入" class="Bool (严格)"("Visible"=w2114) -> ()  [unwired: 2 in, 2 out]
            n1825 = property on="全部读取" class="Bool (严格)"("Visible"=w2113) -> ()  [unwired: 2 in, 2 out]
            n1826 = property on="从板号" class="DigNum (严格)"("Visible"=w2111) -> ()  [unwired: 2 in, 2 out]
            n1827 = local write "主从选择"(w2125) -> ()
            n1828 = property on="从板个数" class="DigNum (严格)"("Visible"=w2117) -> ()  [unwired: 2 in, 2 out]
            n1829 = for {
              tunnel: u32 87470 -> [w2129]
              tunnel: w2122 -> [w2128] mode=indexing
              n1830 = property class="Bool (严格)"(reference=w2128, "BoolText.TextColor"=w2129) -> ()  [unwired: 1 in, 2 out]
            }
            n1831 = Not(x=w2117) -> (.not. x?=w2118:bool)
            n1832 = property class="Bool (严格)"(reference=w2121, "BoolText.TextColor"=u32 16777215) -> ()  [unwired: 1 in, 2 out]
            n1833 = property on="主板选项" class="Tree (严格)"("Visible"=w2117) -> ()  [unwired: 2 in, 2 out]
            n1834 = property on="从板选项" class="Tree (严格)"("Visible"=w2118) -> ()  [unwired: 2 in, 2 out]
            n1835 = property on="当前从板板号" class="DigNum (严格)"("Visible"=w2118) -> ()  [unwired: 2 in, 2 out]
            n1836 = property on="单个读取" class="Bool (严格)"("Visible"=w2112) -> ()  [unwired: 2 in, 2 out]
            n1837 = property on="单个写入" class="Bool (严格)"("Visible"=w2112) -> ()  [unwired: 2 in, 2 out]
          }
          event "从板号": Value Change {
            n1838 = event-data() -> ()  [unwired: 7 out]
            n1839 = local read "key names"() -> (w2217:string[])
            n1840 = Empty Array?(array=w2217) -> (empty?=w2216:bool)
            n1841 = case shown="假" w2216 {
              tunnel: w2217 -> [w2220 _]
              frame False {
                n1842 = stacked-sequence {
                  seq-local: [w2221 _] -> [_ w2284]
                  tunnel: w2220 -> [w2229 _]
                  frame #0 {
                    w2260 = 2 ("长度")
                    w2257 = 20 ("长度")
                    w2245 = 1 ("索引")
                    n1843 = local read "从板号"() -> (w2221:u8)
                    n1844 = local read "输出数组"() -> (w2230:string[][])
                    n1845 = Decrement(x=w2221) -> (x-1=w2227:u8)
                    n1846 = Index Array(array=w2230, index (col)=w2227) -> (element=w2258:string[])  [unwired: 1 in]
                    n1847 = global write "读配置文件全局2.vi" "从板板号"(w2221) -> ()
                    n1848 = Search 1D Array(1D array=w2229, element="风机开启温度" ("元素")) -> (index of element=w2242:i32)  [unwired: 1 in]
                    n1849 = Search 1D Array(1D array=w2229, element="电压过高一级" ("元素"), start index (0)=w2242) -> (index of element=w2240:i32)
                    n1850 = Decrement(x=w2242) -> (x-1=w2244:i32)
                    n1851 = Array Subset(array=w2258, index=w2245, length=w2244) -> (w2228:string[])
                    n1852 = Array Subset(array=w2258, index=w2240, length=21 ("长度")) -> (w2232:string[])
                    n1853 = Array Subset(array=w2229, index=w2245, length=w2244) -> (w2275:string[])
                    n1854 = Array Subset(array=w2258, index=w2242, length=7 ("长度")) -> (w2238:string[])
                    n1855 = for {
                      tunnel: w2232 -> [w2277] mode=indexing
                      tunnel: [w2276] -> w2231 mode=indexing
                      n1856 = Fract/Exp String To Number(string=w2277) -> (number=w2276:dbl)  [unwired: 3 in, 1 out]
                    }
                    n1857 = for {
                      tunnel: w2238 -> [w2279] mode=indexing
                      tunnel: [w2278] -> w2222 mode=indexing
                      n1858 = Fract/Exp String To Number(string=w2279) -> (number=w2278:dbl)  [unwired: 3 in, 1 out]
                    }
                    n1859 = Delete From Array(array=w2231, length=7 ("长度"), index=0 ("索引")) -> (deleted portion=w2225:dbl[], array with subset deleted=w2235:dbl[])
                    n1860 = Array To Cluster(array=w2222) -> (cluster=w2247:T20)
                    n1861 = global write "读配置文件全局2.vi" "加热控制参数"(w2222) -> ()
                    n1862 = Delete From Array(array=w2235, length=7 ("长度"), index=0 ("索引")) -> (deleted portion=w2224:dbl[], array with subset deleted=w2223:dbl[])
                    n1863 = local write "加热控制参数"(w2247) -> ()
                    n1864 = Array To Cluster(array=w2225) -> (cluster=w2272:T20)
                    n1865 = Array To Cluster(array=w2223) -> (cluster=w2274:T20)
                    n1866 = Array To Cluster(array=w2224) -> (cluster=w2273:T20)
                    n1867 = global write "读配置文件全局2.vi" "三级故障阀值"(w2223) -> ()
                    n1868 = global write "读配置文件全局2.vi" "一级故障阀值"(w2225) -> ()
                    n1869 = global write "读配置文件全局2.vi" "二级故障阀值"(w2224) -> ()
                    n1870 = local write "一级故障 6"(w2272) -> ()
                    n1871 = local write "一级故障 8"(w2274) -> ()
                    n1872 = local write "一级故障 7"(w2273) -> ()
                    n1873 = Search 1D Array(1D array=w2275, element="温度个数" ("元素")) -> (index of element=w2254:i32)  [unwired: 1 in]
                    n1874 = Search 1D Array(1D array=w2275, element="第一个保险通道" ("元素")) -> (index of element=w2255:i32)  [unwired: 1 in]
                    n1875 = Search 1D Array(1D array=w2275, element="电压个数" ("元素")) -> (index of element=w2253:i32)  [unwired: 1 in]
                    n1876 = Search 1D Array(1D array=w2275, element="第1通道电压个数" ("元素")) -> (index of element=w2256:i32)  [unwired: 1 in]
                    n1877 = Array Subset(array=w2228, index=w2253, length=2 ("长度")) -> (w2261:string[])
                    n1878 = Array Subset(array=w2228, index=w2254, length=w2260) -> (w2263:string[])
                    n1879 = Array Subset(array=w2228, index=w2255, length=20 ("长度")) -> (w2264:string[])
                    n1880 = Array Subset(array=w2228, index=w2256, length=w2257) -> (w2262:string[])
                    n1881 = Insert Into Array(array=w2261, new element #1=w2262, new element #2=w2263, new element #3=w2264) -> (w2226:string[])  [unwired: 1 in]
                    n1882 = Array Subset(array=w2275, index=w2253, length=w2260) -> (w2265:string[])
                    n1883 = Array Subset(array=w2275, index=w2254, length=w2260) -> (w2267:string[])
                    n1884 = Array Subset(array=w2275, index=w2255, length=w2257) -> (w2268:string[])
                    n1885 = Array Subset(array=w2275, index=w2256, length=w2257) -> (w2266:string[])
                    n1886 = global write "读配置文件全局2.vi" "表格"(w2226) -> ()
                    n1887 = Insert Into Array(array=w2265, new element #1=w2266, new element #2=w2267, new element #3=w2268) -> (w2270:string[])  [unwired: 1 in]
                    n1888 = Build Array(w2270, w2226) -> (w2269:string[][])
                    n1889 = Transpose 2D Array(2D array=w2269) -> (transposed array=w2271:string[][])
                    n1890 = local write "项目信息 2"(w2271) -> ()
                  }
                  frame #1 {
                    n1891 = Number To Decimal String(number=w2284) -> (decimal integer string=w2282:string)  [unwired: 1 in]
                    n1892 = control-ref of="结果"() -> (w2287:refnum<vi>)
                    n1893 = Concatenate Strings("从板", w2282, "导入完成") -> (w2280:string)
                    n1894 = Build Array(w2280) -> (w2285:string[])
                    n1895 = call "表格编辑.vi"("新元素/子数组"=w2285, "活动单元格:单元格背景色"=u32 6618880, "MCListbox引用句柄"=w2287) -> ()  [unwired: 9 out]
                  }
                }
              }
              frame True {
              }
            }
          }
          event "读配置文件": Value Change {
